vi "Turtlesim Publish.vi"() -> ()   [LabVIEW 2012]
uses:
  <userlib>/ROS for LabVIEW Software/ROS/Code/Console/Servers/ServerSubs/TopicDef.ctl
  <userlib>/ROS for LabVIEW Software/ROS/Code/SubVIs/_ROSDirection.ctl
panel:
  in  "Twist":T1
  out "error out":errorcluster
  in  "stop":bool
  # "This VI is meant to be used with the turtlesim example in ROS. Before running this VI, follow the instructions at http://wiki.ros.org/ROS/Tutorials/UnderstandingTopics"
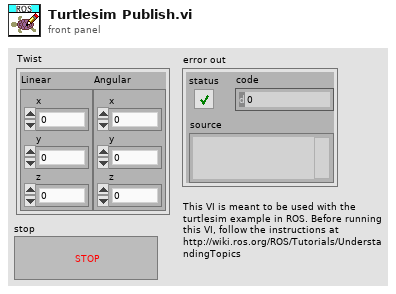
[diagram p1: front panel]
types:
  T1 = cluster{"Linear":cluster{"x":dbl, "y":dbl, "z":dbl}, "Angular":cluster{"x":dbl, "y":dbl, "z":dbl}}
  T2 = typedef "TopicDef.ctl" = cluster{"Topic":string, "Type":string, "Action":T3, "Update (ms)":u16, "queue size":u16}
  T3 = typedef "_ROSDirection.ctl" = enum16{"Node", "Publisher", "Subscriber", "ServiceClient", "ServiceProvider"}
  T4 = typedef "_ROSControl.ctl" = cluster{"topic port":u16, "Node":string, "topic":string, "type":string, "node port":u16, "error ":errorcluster, "Direction":T3, "Update (ms)":u16, "FIFO size":u16}
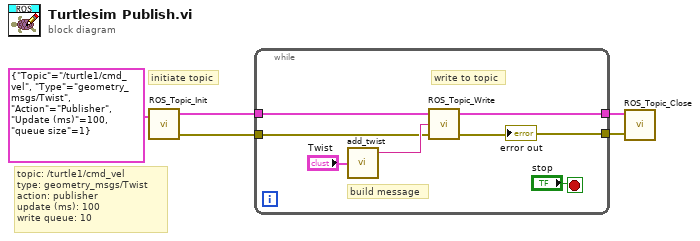
[diagram p0: block diagram]
diagram:
  # "initiate topic"
  # "topic: /turtle1/cmd_vel\ntype: geometry_msgs/Twist\naction: publisher\nupdate (ms): 100\nwrite queue: 10"
  n1 = call <userlib>:"ROS_Topic_Init.vi"("Definitions"=T2 {"Topic"="/turtle1/cmd_vel", "Type"="geometry_msgs/Twist", "Action"=enum."Publisher", "Update (ms)"=100, "queue size"=1}) -> ("ROS out"=w4:T4, "error out"=w3:errorcluster)  [unwired: 2 in]
  n2 = while {
    tunnel: w4 -> [w12]
    tunnel: w3 -> [w10]
    tunnel: [w8] -> w2
    tunnel: [w7] -> w1
    stop <- "stop" stop-if-true
    # "build message"
    # "write to topic"
    n3 = call <userlib>:"add_twist.vi"("Twist"="Twist") -> ("msg out"=w11:string)  [unwired: 4 in]
    n4 = call <userlib>:"ROS_Topic_Write.vi"("error in (no error)"=w10, "Msg in"=w11, "ROS in"=w12) -> ("error out"=w7:errorcluster, "ROS out"=w8:T4)  [unwired: 1 in]
    "error out" <- w7
  }
  n5 = call <userlib>:"ROS_Topic_Close.vi"("error in"=w1, "ROS in"=w2) -> ()  [unwired: 2 in, 1 out]
